vi "HMI Main.vi"() -> ()   [LabVIEW 2011]
uses:
  <vilib>/dex/Flush And Wait Empty Condition.ctl
panel:
  in  "Recipe":T1(array[cluster])=[{"Temp Setpoint"=26.0, "pH Setpoint"=1.7, "Agitation ON"=TRUE, "Intake ON"=FALSE, "Waste ON"=TRUE, "Time (s)"=5.0}, {"Temp Setpoint"=30.0, "pH Setpoint"=1.3, "Agitation ON"=TRUE, "Intake ON"=TRUE, "Waste ON"=FALSE, "Time (s)"=5.0}, {"Temp Setpoint"=27.0, "pH Setpoint"=1.5, "Agitation ON"=FALSE, "Intake ON"=TRUE, "Waste ON"=TRUE, "Time (s)"=5.0}]
  in  "error in":errorcluster
  out "Waste ON":bool
  out "Intake ON":bool
  out "Agitation ON":bool
  in  "Abort Recipe":bool
  out "error out":errorcluster
  in  "Target IP Address":string="10.0.60.140"
  in  "Exit":bool
  in  "Run":bool
  in  "pH Override":bool
  in  "Temp Override":bool
  out "pH":dbl=1420.3838074568646
  in  "pH Setpoint":dbl
  out "Temp":dbl=25.939344155359862
  in  "Temp Setpoint":dbl
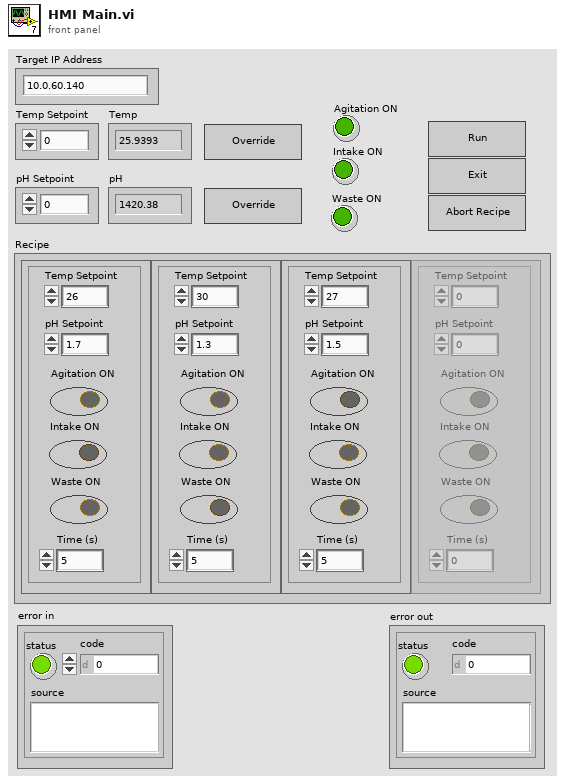
[diagram p1: front panel]
types:
  T1 = cluster{"Temp Setpoint":dbl, "pH Setpoint":dbl, "Agitation ON":bool, "Intake ON":bool, "Waste ON":bool, "Time (s)":dbl}[]
  T2 = typedef "Flush And Wait Empty Condition.ctl" = u8
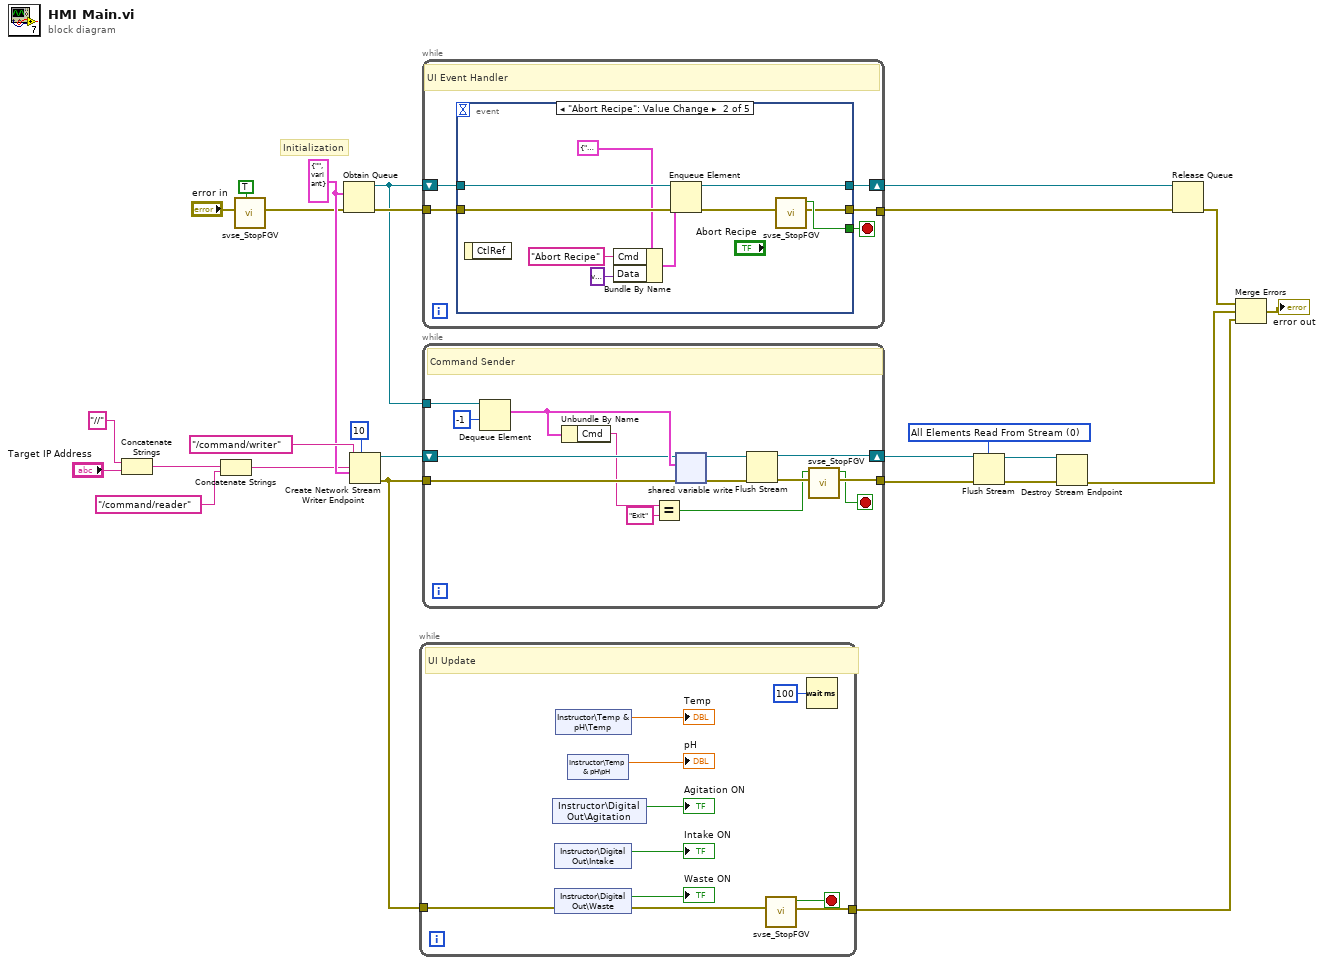
[diagram p0: block diagram]
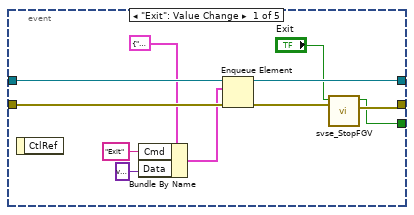
[diagram p2: hidden frame]
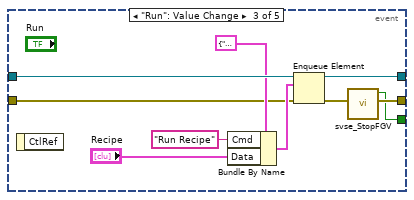
[diagram p3: hidden frame]
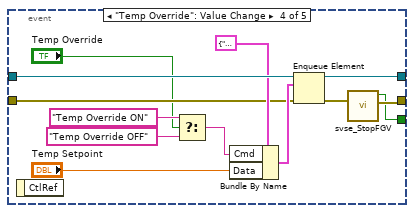
[diagram p4: hidden frame]
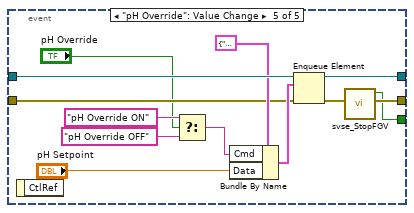
[diagram p5: hidden frame]
diagram:
  w1 = T2 0 items=["All Elements Read From Stream", "All Elements Available for Reading"] ("wait condition")
  w22 = cluster{"Cmd":string, "Data":variant} {"Cmd"="", "Data"=variant}
  # "Initialization"
  n1 = Concatenate Strings("//" ("reader url"), "Target IP Address") -> (w19:string)
  n2 = Concatenate Strings(w19, "/command/reader" ("reader url")) -> (w17:string)
  n3 = call "svse_StopFGV.vi"("Reset (F)"=TRUE, "error in"="error in") -> ("error out"=w10:errorcluster)  [unwired: 8 in, 1 out]
  n4 = Obtain Queue(element data type=w22, error in (no error)=w10) -> (queue out=w25:refnum<queue>, error out=w26:errorcluster)  [unwired: 3 in, 1 out]
  n5 = Create Network Stream Writer Endpoint(7:10 ("writer buffer size"), 9:w22, 10:w17, 11:"/command/writer" ("writer name")) -> (0:w13:errorcluster, 3:w23:refnum<k21>)  [unwired: 2 in]
  n6 = while {
    tunnel: w13 -> [w31]
    tunnel: [w28] -> w12
    stop <- w29 stop-if-true
    # "UI Update"
    n7 = shared-variable "Instructor\\Digital Out\\Agitation"() -> (→"Agitation ON":bool)  [unwired: 1 in, 1 out]
    n8 = shared-variable "Instructor\\Digital Out\\Intake"() -> (→"Intake ON":bool)  [unwired: 1 in, 1 out]
    n9 = shared-variable "Instructor\\Digital Out\\Waste"(error in=w31) -> (→"Waste ON":bool, error out=w30:errorcluster)
    n10 = shared-variable "Instructor\\Temp & pH\\Temp"() -> (→"Temp":dbl)  [unwired: 1 in, 1 out]
    n11 = shared-variable "Instructor\\Temp & pH\\pH"() -> (→"pH":dbl)  [unwired: 1 in, 1 out]
    n12 = call "svse_StopFGV.vi"("error in"=w30) -> ("error out"=w28:errorcluster, "Stop?"=w29:bool)  [unwired: 9 in]
    n13 = Wait (ms)(milliseconds to wait=u32 100) -> ()  [unwired: 1 out]
  }
  n14 = while {
    shift-right: [w37] -> w8
    shift-left: w25 -> [w40]
    tunnel: w26 -> [w39]
    tunnel: [w38] -> w7
    stop <- w41 stop-if-true
    # "UI Event Handler"
    n15 = event shown="[1] \"Abort Recipe\": Value Change" {
      selector: _ -> [_ _ _ _ _]
      dyn-events: _ -> [_ _ _ _ _]
      timeout: _ -> [_ _ _ _ _]
      tunnel: [w42 w54 w64 w73 w86] -> w41
      tunnel: w40 -> [w52 w62 w72 w85 w98]
      tunnel: w39 -> [w50 w60 w67 w80 w94]
      tunnel: [w45 w53 w65 w74 w87] -> w38
      tunnel: [w51 w61 w68 w82 w95] -> w37
      event "Exit": Value Change {
        n16 = event-data() -> ()  [unwired: 1 in, 1 out]
        n17 = Bundle By Name(cluster=cluster{"Cmd":string, "Data":variant} {"Cmd"="", "Data"=variant}, "Cmd"="Exit", "Data"=variant) -> (w47:cluster{"Cmd":string, "Data":variant})
        n18 = Enqueue Element(queue=w52, element=w47, error in (no error)=w50) -> (queue out=w51:refnum<queue>, error out=w44:errorcluster)  [unwired: 1 in, 1 out]
        n19 = call "svse_StopFGV.vi"("error in"=w44, "User stop? (F)"="Exit") -> ("error out"=w45:errorcluster, "Stop?"=w42:bool)  [unwired: 8 in]
      }
      event "Abort Recipe": Value Change {
        n20 = event-data() -> ()  [unwired: 1 in, 1 out]
        n21 = Bundle By Name(cluster=cluster{"Cmd":string, "Data":variant} {"Cmd"="", "Data"=variant}, "Cmd"="Abort Recipe", "Data"=variant) -> (w57:cluster{"Cmd":string, "Data":variant})
        n22 = Enqueue Element(queue=w62, element=w57, error in (no error)=w60) -> (queue out=w61:refnum<queue>, error out=w55:errorcluster)  [unwired: 1 in, 1 out]
        n23 = call "svse_StopFGV.vi"("error in"=w55) -> ("error out"=w53:errorcluster, "Stop?"=w54:bool)  [unwired: 9 in]
      }
      event "Run": Value Change {
        n24 = event-data() -> ()  [unwired: 1 in, 1 out]
        n25 = Bundle By Name(cluster=cluster{"Cmd":string, "Data":variant} {"Cmd"="", "Data"=variant}, "Cmd"="Run Recipe", "Data"="Recipe") -> (w70:cluster{"Cmd":string, "Data":variant})
        n26 = Enqueue Element(queue=w72, element=w70, error in (no error)=w67) -> (queue out=w68:refnum<queue>, error out=w66:errorcluster)  [unwired: 1 in, 1 out]
        n27 = call "svse_StopFGV.vi"("error in"=w66) -> ("error out"=w65:errorcluster, "Stop?"=w64:bool)  [unwired: 9 in]
      }
      event "Temp Override": Value Change {
        n28 = event-data() -> ()  [unwired: 1 in, 1 out]
        n29 = Select(t="Temp Override ON" ("Cmd"), s="Temp Override", f="Temp Override OFF" ("Cmd")) -> (s? t:f=w76:string)
        n30 = Bundle By Name(cluster=cluster{"Cmd":string, "Data":variant} {"Cmd"="", "Data"=variant}, "Cmd"=w76, "Data"="Temp Setpoint") -> (w83:cluster{"Cmd":string, "Data":variant})
        n31 = Enqueue Element(queue=w85, element=w83, error in (no error)=w80) -> (queue out=w82:refnum<queue>, error out=w75:errorcluster)  [unwired: 1 in, 1 out]
        n32 = call "svse_StopFGV.vi"("error in"=w75) -> ("error out"=w74:errorcluster, "Stop?"=w73:bool)  [unwired: 9 in]
      }
      event "pH Override": Value Change {
        n33 = event-data() -> ()  [unwired: 1 in, 1 out]
        n34 = Select(t="pH Override ON" ("Cmd"), s="pH Override", f="pH Override OFF" ("Cmd")) -> (s? t:f=w91:string)
        n35 = Bundle By Name(cluster=cluster{"Cmd":string, "Data":variant} {"Cmd"="", "Data"=variant}, "Cmd"=w91, "Data"="pH Setpoint") -> (w96:cluster{"Cmd":string, "Data":variant})
        n36 = Enqueue Element(queue=w98, element=w96, error in (no error)=w94) -> (queue out=w95:refnum<queue>, error out=w88:errorcluster)  [unwired: 1 in, 1 out]
        n37 = call "svse_StopFGV.vi"("error in"=w88) -> ("error out"=w87:errorcluster, "Stop?"=w86:bool)  [unwired: 9 in]
      }
    }
  }
  n38 = while {
    tunnel: w25 -> [w112]
    shift-right: [w104] -> w6
    shift-left: w23 -> [w109]
    tunnel: w13 -> [w107]
    tunnel: [w101] -> w5
    stop <- w100 stop-if-true
    # "Command Sender"
    n39 = Dequeue Element(queue=w112, timeout in ms (-1)=-1) -> (element=w110:cluster{"Cmd":string, "Data":variant})  [unwired: 1 in, 3 out]
    n40 = Unbundle By Name(w110) -> ("Cmd"=w106:string)
    n41 = Equal?(x=w106, y="Exit") -> (x = y?=w99:bool)
    n42 = shared-variable-write ("Write Single Element to Stream")(w109, w107, w110) -> (w105:refnum<k21>, w103:errorcluster)  [unwired: 1 in, 1 out]
    n43 = Flush Stream(8:w103, 11:w105) -> (0:w102:errorcluster, 3:w104:refnum<k21>)  [unwired: 2 in, 1 out]
    n44 = call "svse_StopFGV.vi"("error in"=w102, "User stop? (F)"=w99) -> ("error out"=w101:errorcluster, "Stop?"=w100:bool)  [unwired: 8 in]
  }
  n45 = Flush Stream(8:w5, 10:w1, 11:w6) -> (0:w3:errorcluster, 3:w4:refnum<k21>)  [unwired: 1 in, 1 out]
  n46 = Destroy Stream Endpoint(8:w3, 11:w4) -> (0:w2:errorcluster)
  n47 = Release Queue(queue=w8, error in (no error)=w7) -> (error out=w15:errorcluster)  [unwired: 1 in, 2 out]
  n48 = Merge Errors(w15, w2, w12) -> (→"error out":errorcluster)
